vi "PH_PPMA_PowerUnit.set modified data.vi"(0 "i ref in":refnum<vi>, 2 "i attribute":T1={"GUI Refs"={"Rods"=refnum, "Ignitron"=refnum, "Rossrelais"=refnum, "Set Voltage"=refnum, "PSU"=refnum, "EOC"=refnum, "Trigger"=refnum}, "Rods"={"Instancename"="N/A", "Device Status"=-1, "linked?"=FALSE}, "PSU"={"lower limit [V]"=0.0, "upper limit [V]"=0.0, "Voltage set"=FALSE, "State Device"=0, "linked?"=FALSE}, "Ross Relais"={"State Device"=0, "linked?"=FALSE}, "Ignitron"={"State Device"=0, "linked?"=FALSE}, "Trigger"={"State Device"=0, "linked?"=FALSE}, "Timing Settings"={"Prdc Fast?"=FALSE, "Default Value Periodic Interval"=0, "Mercury on since"=30.0, "Warm up Time Mercury [s]"=9999.0}, "Set Voltage [V]"=0.0} {"Trigger"."State Device" items=["no info", "off/false/out", "on/true/in", "Failure", "Alarm", "Status 1", "Status 2", "Status 3"]; "Ignitron"."State Device" items=["no info", "off/false/out", "on/true/in", "Failure", "Alarm", "Status 1", "Status 2", "Status 3"]; "Ross Relais"."State Device" items=["no info", "off/false/out", "on/true/in", "Failure", "Alarm", "Status 1", "Status 2", "Status 3"]; "PSU"."State Device" items=["no info", "off/false/out", "on/true/in", "Failure", "Alarm", "Status 1", "Status 2", "Status 3"]; "Rods"."Device Status" items=["no info", "off/false/out", "on/true/in", "Failure", "Alarm", "Status 1", "Status 2", "Status 3"]}, 5 "error in (no error)":errorcluster) -> (14 "i ref out":refnum<vi>, 19 "error out":errorcluster)   [LabVIEW 2014, in "PH_PPMA_PowerUnit.lvlib"]
doc: "Writes the data into the attribute of an object. Then, the attribute dara are unlocked using the \"release\" method. Prior to calling THIS method, the attribute data must have been locked using the methods \"lock\" or \"get data to modify\".\n\n\nLicense Agreement for this software:\n\nCopyright (C)\nGesellschaft für Schwerionenforschung, GSI\nPlanckstr. 1\n64291 Darmstadt\nGermany\n\nContact: D.Beck@gsi.de \n\nThis program is free software; you can redistribute it and/or modify it under the terms of the GNU General Public License as published by the Free Software Foundation; either version 2 of the license, or (at your option) any later version.\n\nThis program is distributed in the hope that it will be useful, but WITHOUT ANY WARRANTY; without even the implied warranty of MERCHANTABILITY or FITNESS FOR A PARTICULAR PURPOSE. See the GNU General License for more details (http://www.gnu.org).\n\nGesellschaft für Schwerionenforschung, GSI\nPlanckstr. 1, 64291 Darmstadt, Germany\nFor all questions and ideas contact: M.Richter@gsi.de, H.Brand@gsi.de or D.Beck@gsi.de.\nLast update: 17-JUN-2004"
uses:
  PH_PPMA_PowerUnit.lvlib
  PH_PPMA_PowerUnit.i attribute.ctl
  PH_PPMA_PowerUnit.Rods Attributes.ctl
  PH_StatusHandler/PH_StatusHandler.Status.ctl
  PH_PP_Common/PH_PP_Common.PSU Attributes.ctl
  PH_PP_Common/PH_PP_Common.Ross Relais Attributes.ctl
  PH_PP_Common/PH_PP_Common.Ignitron Attributes.ctl
  CSCore/CSObj/CSObj.lvlib
  PH_PP_Common/PH_PP_Common.lvlib
  PH_StatusHandler/PH_StatusHandler.lvlib
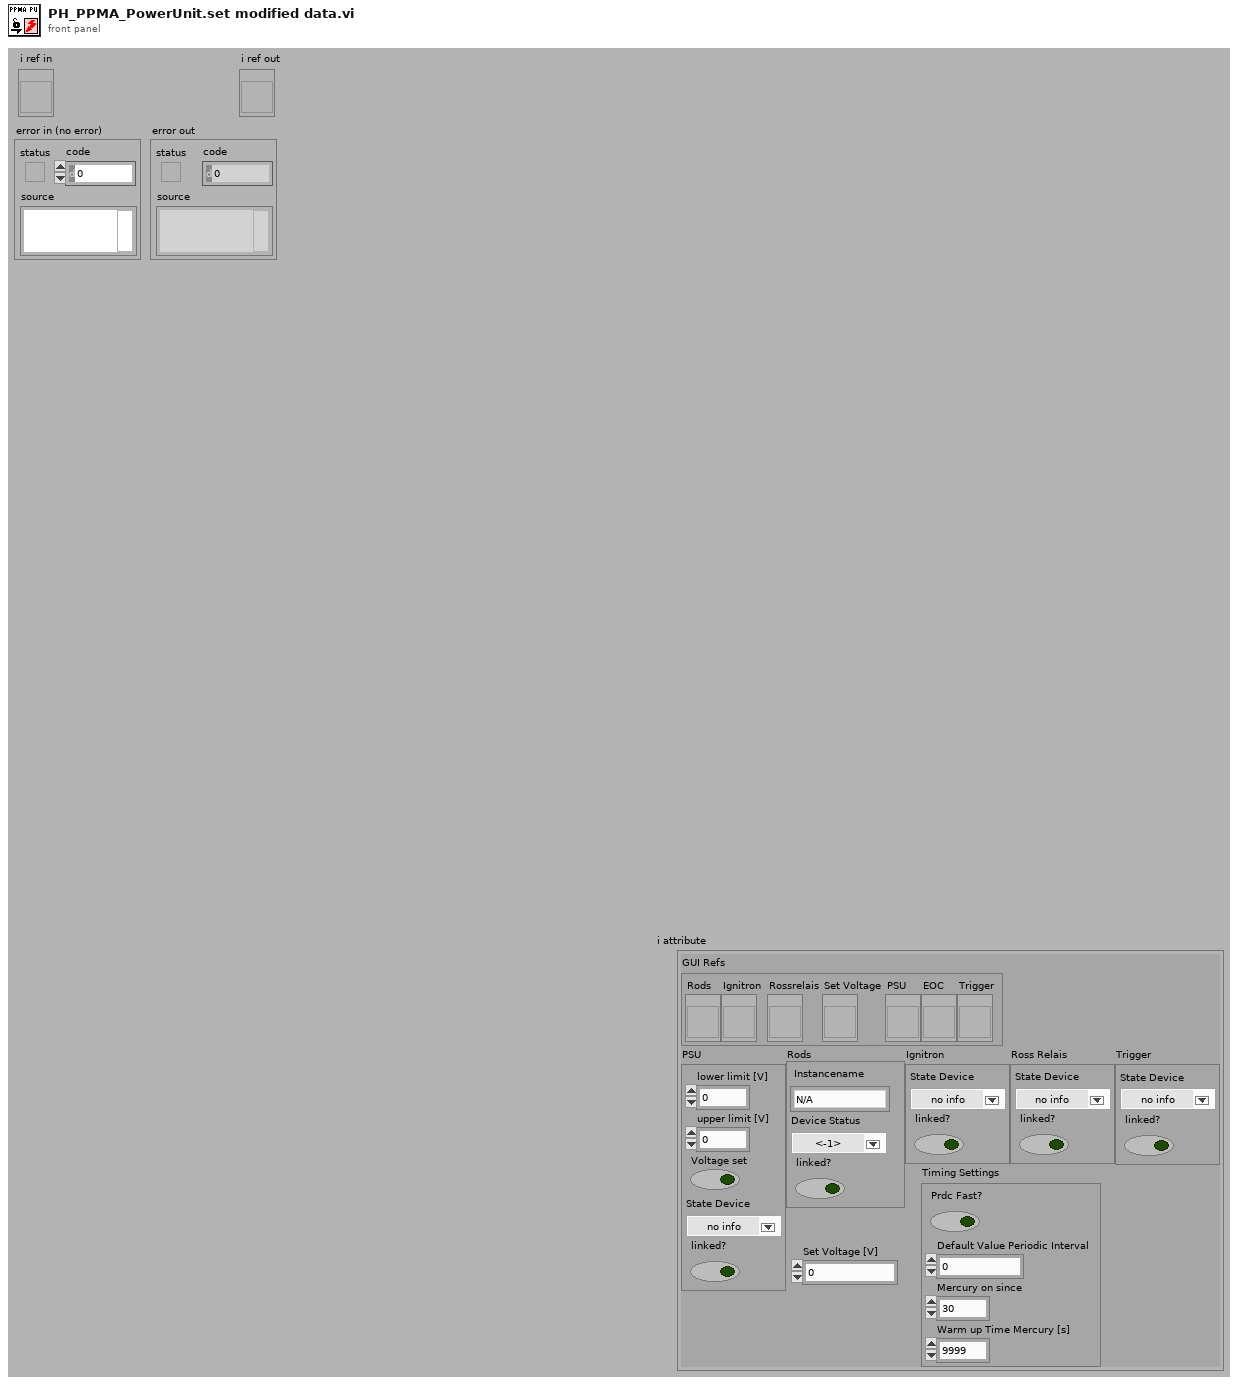
[diagram p1: front panel]
types:
  T1 = typedef "PH_PPMA_PowerUnit.lvlib/PH_PPMA_PowerUnit.i attribute.ctl" = cluster{"GUI Refs":cluster{"Rods":refnum<vi>, "Ignitron":refnum<vi>, "Rossrelais":refnum<vi>, "Set Voltage":refnum<vi>, "PSU":refnum<vi>, "EOC":refnum<vi>, "Trigger":refnum<vi>}, "Rods":T2, "PSU":T4, "Ross Relais":T5, "Ignitron":T6, "Trigger":cluster{"State Device":T3, "linked?":bool}, "Timing Settings":cluster{"Prdc Fast?":bool, "Default Value Periodic Interval":i32, "Mercury on since":dbl, "Warm up Time Mercury [s]":dbl}, "Set Voltage [V]":dbl}
  T2 = typedef "PH_PPMA_PowerUnit.lvlib/PH_PPMA_PowerUnit.Rods Attributes.ctl" = cluster{"Instancename":string, "Device Status":T3, "linked?":bool}
  T3 = typedef "PH_StatusHandler.lvlib/PH_StatusHandler.Status.ctl" = i16
  T4 = typedef "PH_PP_Common.lvlib/PH_PP_Common.PSU Attributes.ctl" = cluster{"lower limit [V]":dbl, "upper limit [V]":dbl, "Voltage set":bool, "State Device":T3, "linked?":bool}
  T5 = typedef "PH_PP_Common.lvlib/PH_PP_Common.Ross Relais Attributes.ctl" = cluster{"State Device":T3, "linked?":bool}
  T6 = typedef "PH_PP_Common.lvlib/PH_PP_Common.Ignitron Attributes.ctl" = cluster{"State Device":T3, "linked?":bool}
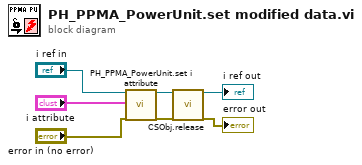
[diagram p0: block diagram]
diagram:
  n1 = call "PH_PPMA_PowerUnit.set i attribute.vi"("i ref in"="i ref in", "i attribute"="i attribute", "error in (no error)"="error in (no error)") -> ("i ref out"=w4:refnum<vi>, "error out"=w3:errorcluster)  [unwired: 15 in]
  n2 = call "CSObj.release.vi"("i ref in"=w4, "error in (no error)"=w3) -> ("i ref out"=→"i ref out":refnum<vi>, "error out"=→"error out":errorcluster)  [unwired: 16 in]
